vi "Pause.vi"(8 "error in (no error)":errorcluster, 11 "Sonicator Module State Cluster":T1={"State"=enum."Idle", "Start Time"=timestamp(0 s since 1904-01-01), "Current Time"=timestamp(0 s since 1904-01-01), "Agitator Module Config"={"GUID"="", "Drop Coords"={"Horizontal"=0, "Vertical"=0}, "Process Name"="", "User name"="", "Queue Name"="", "Settings"={"Cycle Period"=500.0, "Agitator Type"="", "Setpoint (µm)"=0.0, "IKA EUROSTAR Settings"={"VISA resource name"="", "Simulated?"=FALSE}}, "Load Count"=0}, "Output Error"=FALSE, "Log Started"=FALSE, "First Iteration"=FALSE, "Data"={"Agitator rpm Value"=0.0}, "Agitator On?"=enum."Off"}) -> (0 "error out":errorcluster, 3 "Sonicator Module State Cluster":T1={"State"=enum."Idle", "Start Time"=timestamp(0 s since 1904-01-01), "Current Time"=timestamp(0 s since 1904-01-01), "Agitator Module Config"={"GUID"="", "Drop Coords"={"Horizontal"=0, "Vertical"=0}, "Process Name"="", "User name"="", "Queue Name"="", "Settings"={"Cycle Period"=500.0, "Agitator Type"="", "Setpoint (µm)"=0.0, "IKA EUROSTAR Settings"={"VISA resource name"="", "Simulated?"=FALSE}}, "Load Count"=0}, "Output Error"=FALSE, "Log Started"=FALSE, "First Iteration"=FALSE, "Data"={"Agitator rpm Value"=0.0}, "Agitator On?"=enum."Off"})   [LabVIEW 2018, in "Agitator Module.lvlib" / "Agitator Module Engine.lvlib"]
uses:
  Agitator Module Engine.lvlib
  Feed Module/Controls/Agitator Module State Cluster.ctl
  Pump Module Folder/Measure Instrument/State Enum.ctl
  Feed Module/Controls/Agitator Module Config Cluster.ctl
  <vilib>/Utility/miscctls.llb/LVPoint32TypeDef.ctl
  Feed Module/Controls/Agitator Module Settings Cluster.ctl
  IKA EUROSTAR/IKA EUROSTAR Settings.ctl
  Tag VIs/Tag FGV Operation Enum.ctl
  Shared Variables/Dynamic Shared Variables.lvlib
  Sonic Systems P100/Sonic Systems P100.lvlib
  Pump Module Folder/Measure Instrument/Pump Module Engine.lvlib
  Agitator Module.lvlib
  IKA EUROSTAR/IKA EUROSTAR.lvlib
panel:
  # "Agitator Settings"
  # "Agitator Settings"
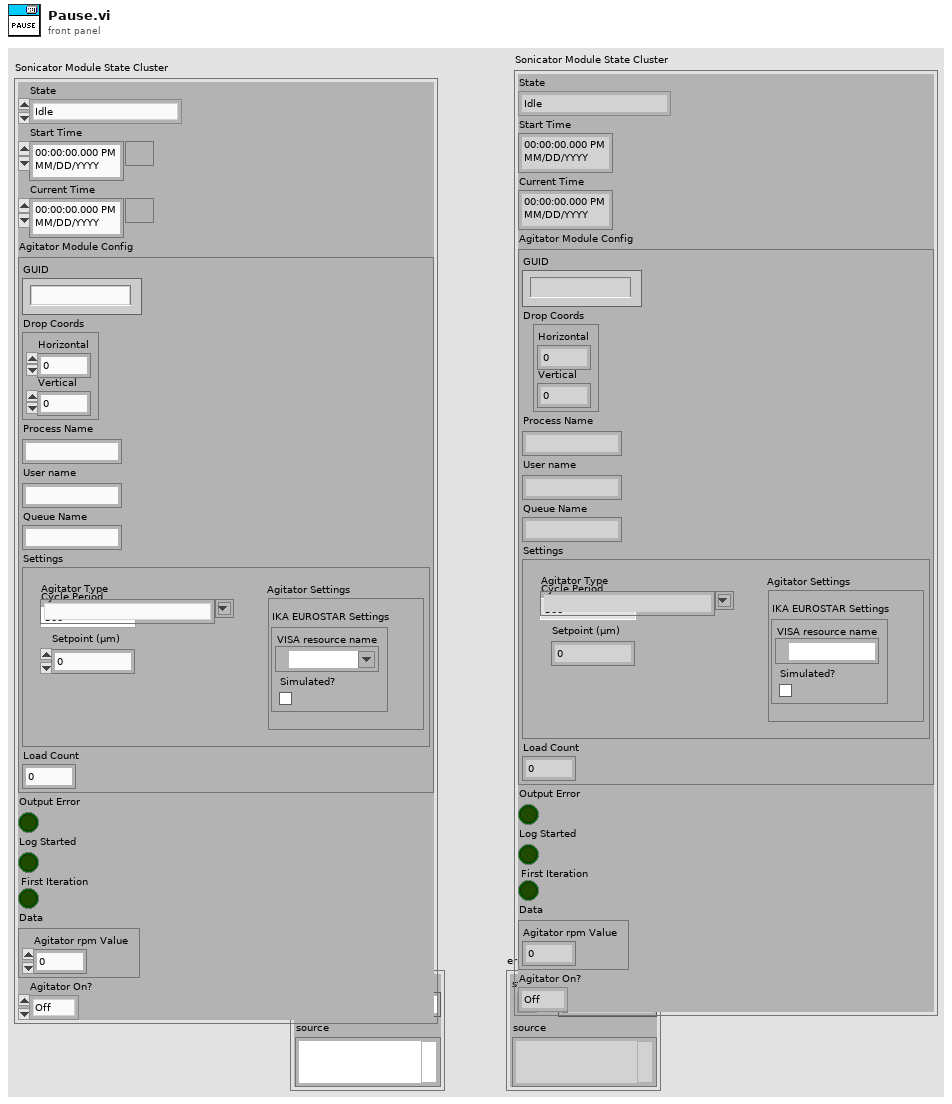
[diagram p1: front panel]
types:
  T1 = typedef "Agitator Module.lvlib/Agitator Module State Cluster.ctl" = cluster{"State":T2, "Start Time":timestamp, "Current Time":timestamp, "Agitator Module Config":T3, "Output Error":bool, "Log Started":bool, "First Iteration":bool, "Data":cluster{"Agitator rpm Value":dbl}, "Agitator On?":enum16{"Off", "On", "Not Initialized", "Over Cutoff"}}
  T2 = typedef "Pump Module.lvlib/Pump Module Engine.lvlib/State Enum.ctl" = enum16{"Measuring", "Idle", "Paused"}
  T3 = typedef "Agitator Module.lvlib/Agitator Module Config Cluster.ctl" = cluster{"GUID":string, "Drop Coords":T4, "Process Name":string, "User name":string, "Queue Name":string, "Settings":T5, "Load Count":i32}
  T4 = typedef "LVPoint32TypeDef.ctl" = cluster{"Horizontal":i32, "Vertical":i32}
  T5 = typedef "Agitator Module.lvlib/Agitator Module Settings Cluster.ctl" = cluster{"Cycle Period":dbl, "Agitator Type":string, "Setpoint (µm)":dbl, "IKA EUROSTAR Settings":T6}
  T6 = typedef "IKA EUROSTAR.lvlib/IKA EUROSTAR Settings.ctl" = cluster{"VISA resource name":refnum<visa-resource-name>, "Simulated?":bool}
  T7 = typedef "Sonic Systems P100.lvlib/Sonic Systems P100 Settings.ctl" = cluster{"VISA resource name":refnum<visa-resource-name>, "Simulated?":bool}
  T8 = cluster{"Amplitude Tag":string, "Power Tag":string, "Output Device Tag":string}
  T9 = typedef "Tag FGV Operation Enum.ctl" = enum16{"Init", "Set Notification Queue", "Create Tag", "Commit", "Write Tag (Numeric)", "Write Tag (Boolean)", "Read All Tags", "Read One Tag", "Delete Tag Category", "Set Alarm Parameters (Numeric)", "Set Alarm Parameters (Boolean)", "Enable All Alarms", "Disable All Alarms", "Delete All Tags", "Read Alarms", "Ack Alarm", "Read Alarm Parameters (Numeric)", "Read Alarm Parameters (Boolean)"}
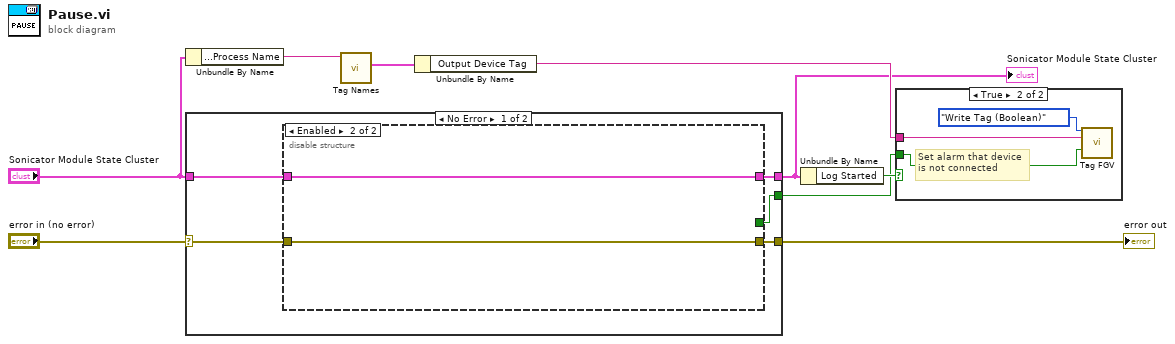
[diagram p0: block diagram]
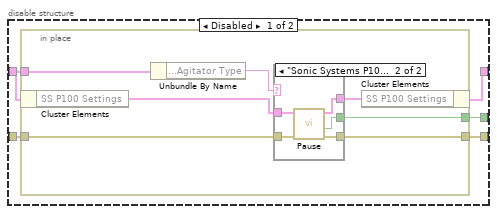
[diagram p3: hidden frame]
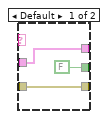
[diagram p4: hidden frame]
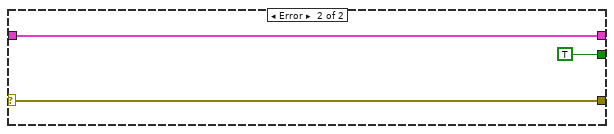
[diagram p5: hidden frame]
diagram:
  n1 = Unbundle By Name("Sonicator Module State Cluster") -> ("Agitator Module Config.Process Name"=w1:string)
  n2 = case shown="No Error" "error in (no error)" {
    selector: "error in (no error)" -> [w13 w39]
    tunnel: [w14 w39] -> w8
    tunnel: "Sonicator Module State Cluster" -> [w10 w38]
    tunnel: [w12 w38] -> w4
    tunnel: [w11 TRUE ("Connection Error")] -> w5
    frame No Error {
      n3 = disable-structure shown="Enabled" {
        disable-tunnel: [w19 w35] -> w14
        disable-tunnel: w13 -> [w18 w35]
        disable-tunnel: [w17 w36] -> w12
        disable-tunnel: [w16 _] -> w11
        disable-tunnel: w10 -> [w15 w36]
        frame Disabled {
          n4 = in-place {
            in-place-border: [w26] -> w19
            in-place-border: w18 -> [w25]
            in-place-border: [w22] -> w16
            in-place-border: w15 -> [w21]
            n5 = in-place-cluster #1(w15) -> ("SS P100 Settings"=w24:T7)
            n6 = Unbundle By Name(w21) -> ("Agitator Module Config.Settings.Agitator Type"=w20:string)
            n7 = case shown="\"Sonic Systems P100\"" w20 {
              tunnel: [w28 w34] -> w26
              tunnel: w25 -> [w28 w33]
              tunnel: w24 -> [w29 w32]
              tunnel: [w29 w31] -> w23
              tunnel: [FALSE ("Connection Error") w30] -> w22
              frame Default {
              }
              frame "Sonic Systems P100" {
                n8 = call "Pause.vi"("error in (no error)"=w33, "SS P100 Settings In"=w32) -> ("error out"=w34:errorcluster, "Connection Error"=w30:bool, "SS P100 Settings Out"=w31:T7)  [unwired: 7 in]
              }
            }
            n9 = in-place-cluster #1("SS P100 Settings"=w23) -> (w17:T1)
          }
        }
        frame Enabled {
        }
      }
    }
    frame Error {
    }
  }
  "error out" <- w8
  "Sonicator Module State Cluster" <- w4
  n10 = call "Tag Names.vi"("Process Name"=w1) -> ("SC Tags"=w3:T8)  [unwired: 8 in, 2 out]
  n11 = Unbundle By Name(w3) -> ("Output Device Tag"=w7:string)
  n12 = Unbundle By Name(w4) -> ("Log Started"=w6:bool)
  n13 = case shown="True" w6 {
    tunnel: w7 -> [_ w41]
    tunnel: w5 -> [_ w40]
    frame False {
    }
    frame True {
      # "Set alarm that device\nis not connected"
      n14 = call "Tag FGV.vi"("Operation"=Tag_FGV_Operation_Enum."Write Tag (Boolean)", "Tag Name"=w41, "Data"=w40) -> ()  [unwired: 5 in, 8 out]
    }
  }
